vi "Set Text Icon on Library.vi"(8 "error in":errorcluster, 11 "reference":refnum<vi>) -> (0 "error out":errorcluster)   [LabVIEW 2020]
uses:
  <vilib>/LabVIEW Icon API/Set Text Icon/Text-Based VI Icon.lvlib
  <vilib>/ProgressBar/Progress Bar Dialog.lvclass
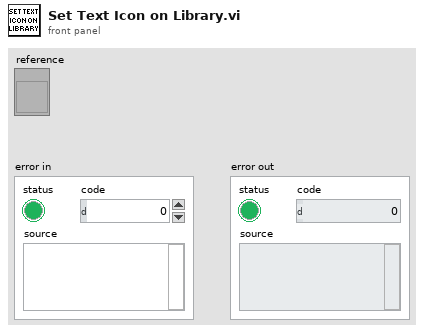
[diagram p1: front panel]
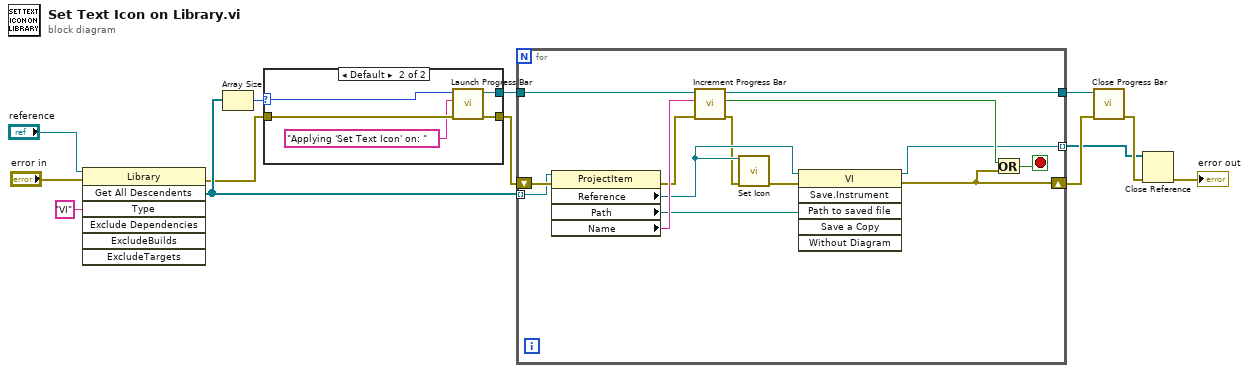
[diagram p0: block diagram]
diagram:
  n1 = invoke class="Library" method="Get All Descendents"(reference="reference", error in="error in", "Type"="VI") -> (error out=w5:errorcluster, "All Descendents"=w10:refnum<vi>[])  [unwired: 4 in, 5 out]
  n2 = Array Size(array=w10) -> (size(s)=w11:i32)
  n3 = case shown="Default" w11 {
    selector: w11 -> [_ w16]
    tunnel: [_ w19] -> w9
    tunnel: w5 -> [w14 w18]
    tunnel: [w14 w17] -> w7
    frame 0 {
    }
    frame Default {
      n4 = call <vilib>:"Launch Progress Bar.vi"("error in (no error)"=w18, "Main Title (\"Working...\")"="Applying 'Set Text Icon' on: " ("Main Title (\"Working...\")"), "Total Count"=w16) -> ("error out"=w17:errorcluster, "Progress Bar Dialog"=w19:refnum<class "Progress Bar Dialog.lvclass">)  [unwired: 7 in]
    }
  }
  n5 = for {
    shift-right: [w20] -> w6
    shift-left: w7 -> [w33]
    tunnel: w10 -> [w32] mode=indexing
    tunnel: w9 -> [w29]
    tunnel: [w28] -> w8
    tunnel: [w22] -> w1 mode=indexing
    stop <- w31 stop-if-true
    n6 = property class="ProjectItem"(reference=w32, error in=w33) -> (error out=w25:errorcluster, "Reference"=w26:refnum<vi>, "Path"=w21:path, "Name"=w27:string)  [unwired: 1 out]
    n7 = call <vilib>:"Increment Progress Bar.vi"("error in (no error)"=w25, "Step Name (\"\")"=w27, "Progress Bar Dialog in"=w29) -> ("error out"=w24:errorcluster, "Cancelled?"=w30:bool, "Progress Bar Dialog out"=w28:refnum<class "Progress Bar Dialog.lvclass">)  [unwired: 6 in]
    n8 = call <vilib>:"Set Icon.vi"("VI"=w26, "error in"=w24) -> ("error out"=w23:errorcluster)  [unwired: 12 in, 1 out]
    n9 = invoke class="VI" method="Save.Instrument"(reference=w26, error in=w23, "Path to saved file"=w21) -> (reference out=w22:refnum<vi>, error out=w20:errorcluster)  [unwired: 3 in, 4 out]
    n10 = Or(x=w30, y=w20) -> (x .or. y?=w31:bool)
  }
  n11 = call <vilib>:"Close Progress Bar.vi"("error in (no error)"=w6, "Progress Bar Dialog"=w8) -> ("error out"=w4:errorcluster)  [unwired: 9 in]
  n12 = Close Reference(reference=w1, error in (no error)=w4) -> (error out=→"error out":errorcluster)
